vi "Write Address List.vi"(8 "error in (no error)":errorcluster, 10 "Address List":u16[](array[numeric]), 11 "1553 SubComponent in":refnum<class "1553 SubComponent.lvclass">) -> (0 "error out":errorcluster, 3 "1553 SubComponent out":refnum<class "1553 SubComponent.lvclass">)   [LabVIEW 2016]
uses:
  1553 SubComponent.lvclass
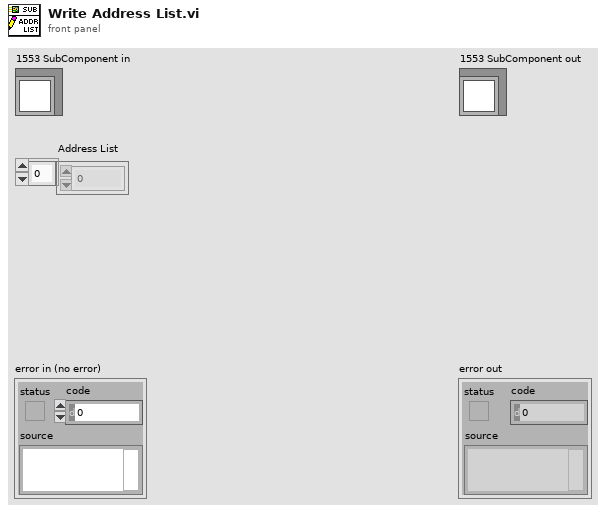
[diagram p1: front panel]
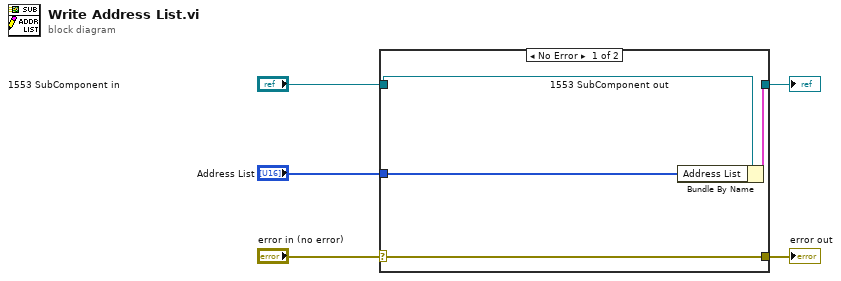
[diagram p0: block diagram]
diagram:
  n1 = case shown="No Error" "error in (no error)" {
    selector: "error in (no error)" -> [w9 w10]
    tunnel: [w9 w10] -> w4
    tunnel: [w7 w11] -> w2
    tunnel: "1553 SubComponent in" -> [w8 w11]
    tunnel: "Address List" -> [w6 _]
    frame No Error {
      n2 = Bundle By Name(cluster=w8, "Address List"=w6) -> (w7:cluster{})
    }
    frame Error {
    }
  }
  "error out" <- w4
  "1553 SubComponent out" <- w2
